vi "TOP-累积剂量数据管理.vi"(8 "错误输出":errorcluster, 11 "DB动作集":T1) -> (0 "error out":errorcluster, 3 "输出数据":variant)   [LabVIEW 2017]
uses:
  <vilib>/addons/database/Connection.llb/Conn ObjectReference.ctl
  <vilib>/addons/database/NI_Database_API.lvlib
panel:
  out "累积记录":T3
  out "探测器信息":T4
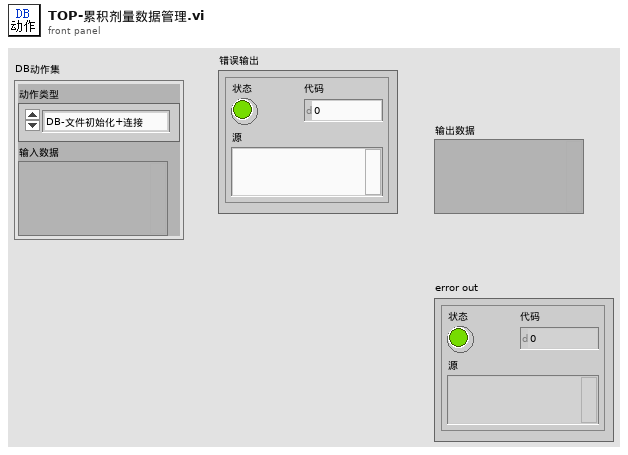
[diagram p1: front panel]
types:
  T1 = typedef "DB动作与数据.ctl" = cluster{"动作类型":T2, "输入数据":variant}
  T2 = typedef "DB动作类型.ctl" = enum16{"DB-文件初始化+连接", "DB-断开连接", "DB-结构初始化", "DB-加载设备", "DB-检查连接状态", "设备-登记新设备+数据表", "设备-删除设备", "设备-修改网址", "设备-修改名称+转移数据", "设备-修改备注", "设备-修改限值", "设备-累积校准", "设备-重排", "数据-获取全部", "数据-删除数据", "数据-写改累积记录+改累积剂量", "读变量-全部设备"}
  T3 = typedef "单条累积记录.ctl" = cluster{"起始时间":timestamp, "结束时间":timestamp, "累积剂量":dbl}
  T4 = typedef "探测器信息.ctl" = cluster{"网络地址":string, "名称":string, "备注":string, "累积剂量":dbl, "累积限值":dbl, "硬件剂量率限值":T5, "剂量率限值1":dbl, "剂量率限值2":dbl, "报警方式":T6}
  T5 = typedef "探头剂量率限值选择.ctl" = enum16{"一级限值", "二级限值"}
  T6 = typedef "报警方式选择.ctl" = enum16{"常报警", "自动静音", "手动静音"}
  T7 = typedef "修改网址.ctl" = cluster{"探头属性":T4, "新网址":string}
  T8 = typedef "设备改名卡.ctl" = cluster{"原名":string, "新名":string}
  T9 = typedef "删除记录输入.ctl" = cluster{"名称":string, "多条记录(空则全删)":T3[]}
  T10 = typedef "写改累积记录输入.ctl" = cluster{"探头地址与信息":T4, "测量值":T11, "累积记录":T3}
  T11 = typedef "测量值.ctl" = cluster{"时间":timestamp, "数值":dbl}
  T12 = typedef "NI_Database_API.lvlib/Conn ObjectReference.ctl" = refnum<k1>
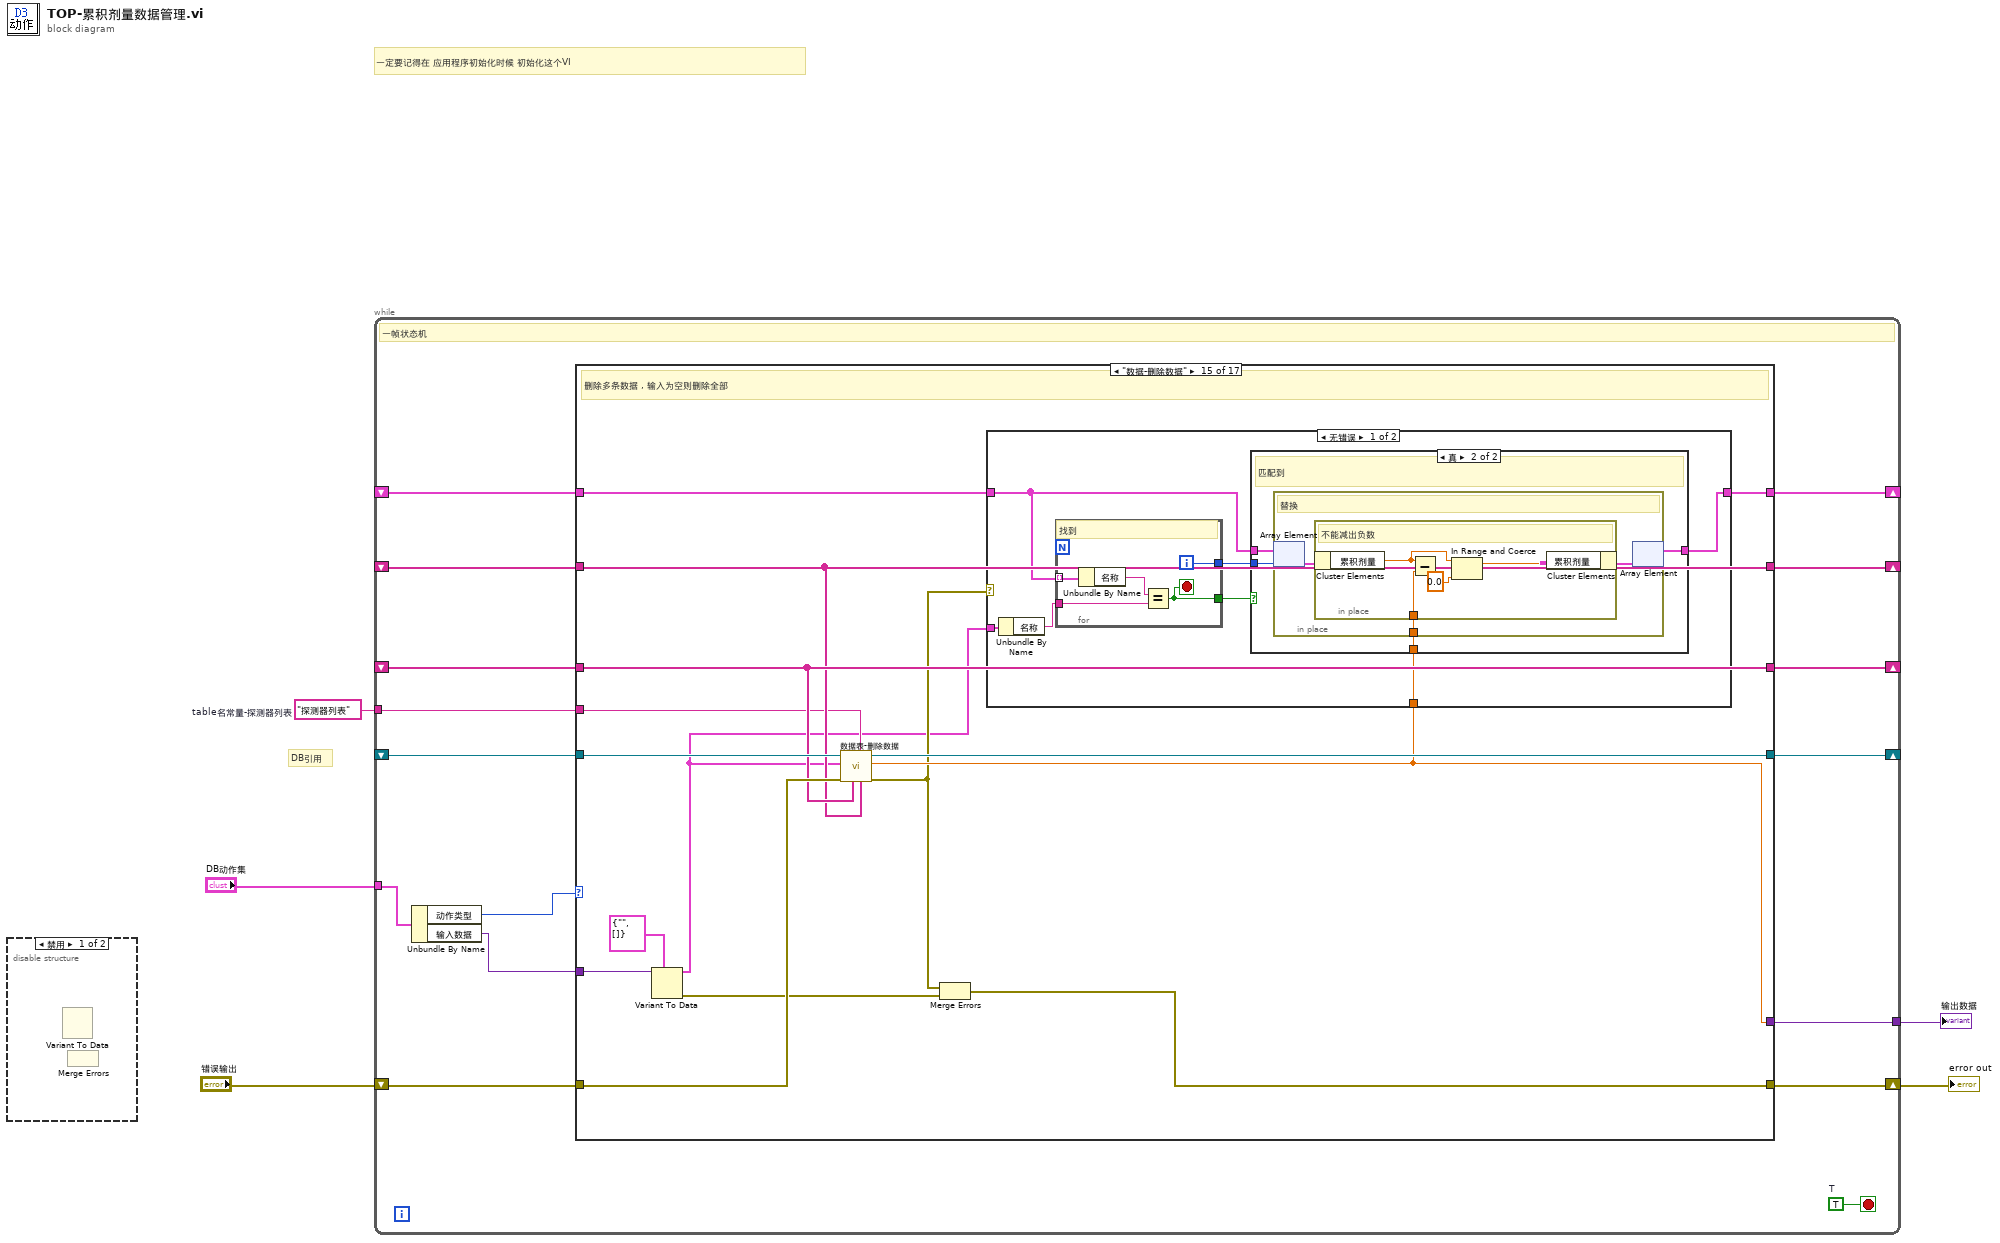
[diagram p0: block diagram]
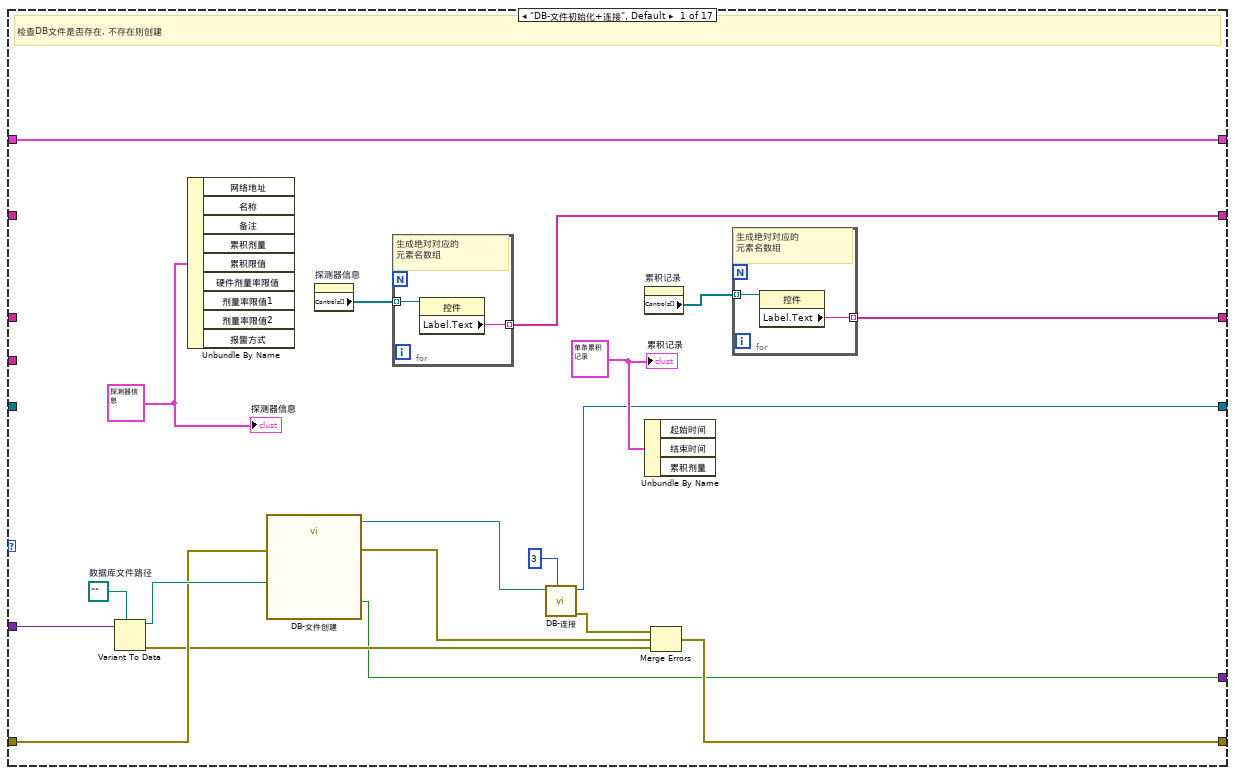
[diagram p3: hidden frame]
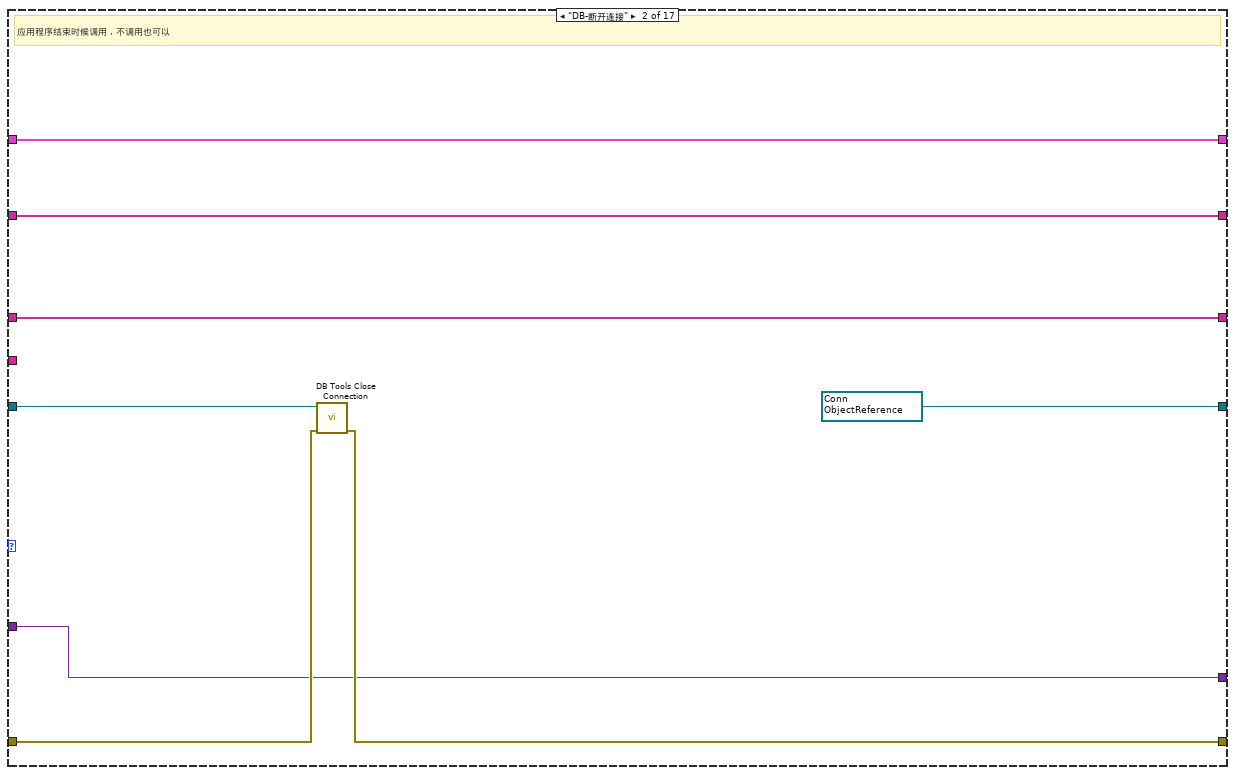
[diagram p4: hidden frame]
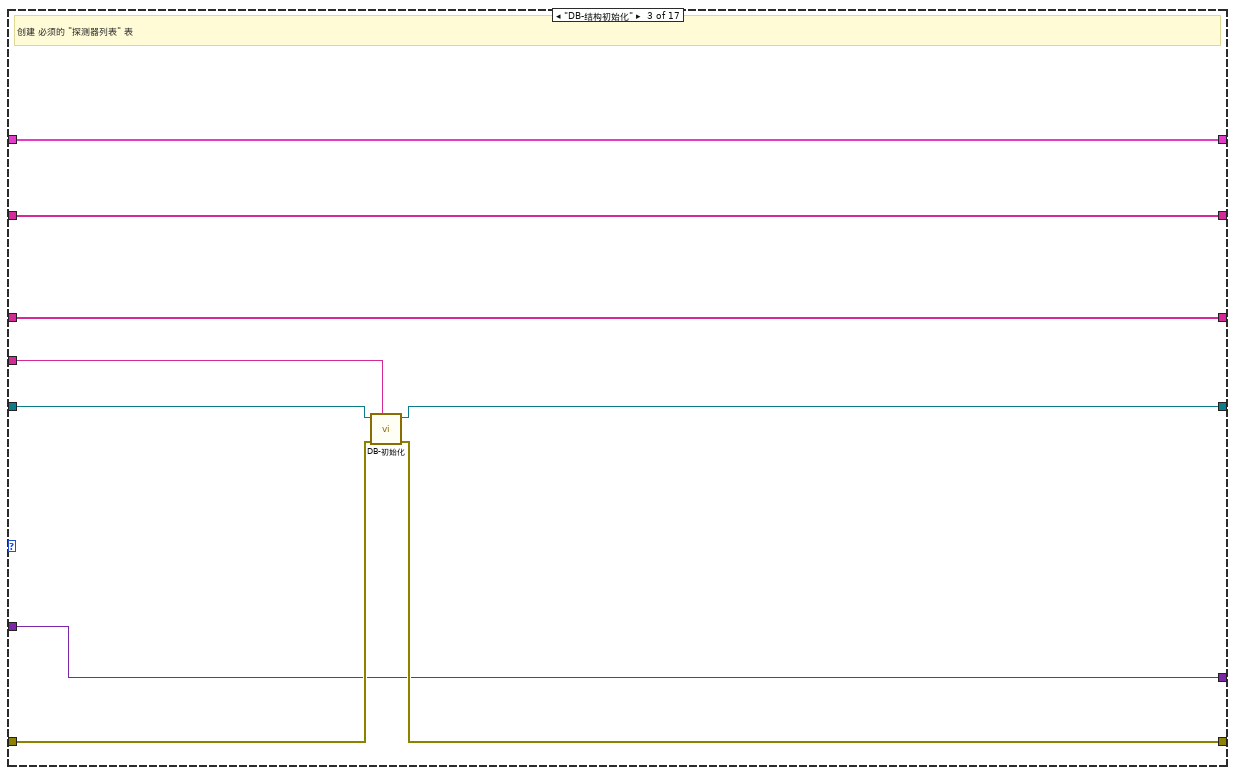
[diagram p5: hidden frame]
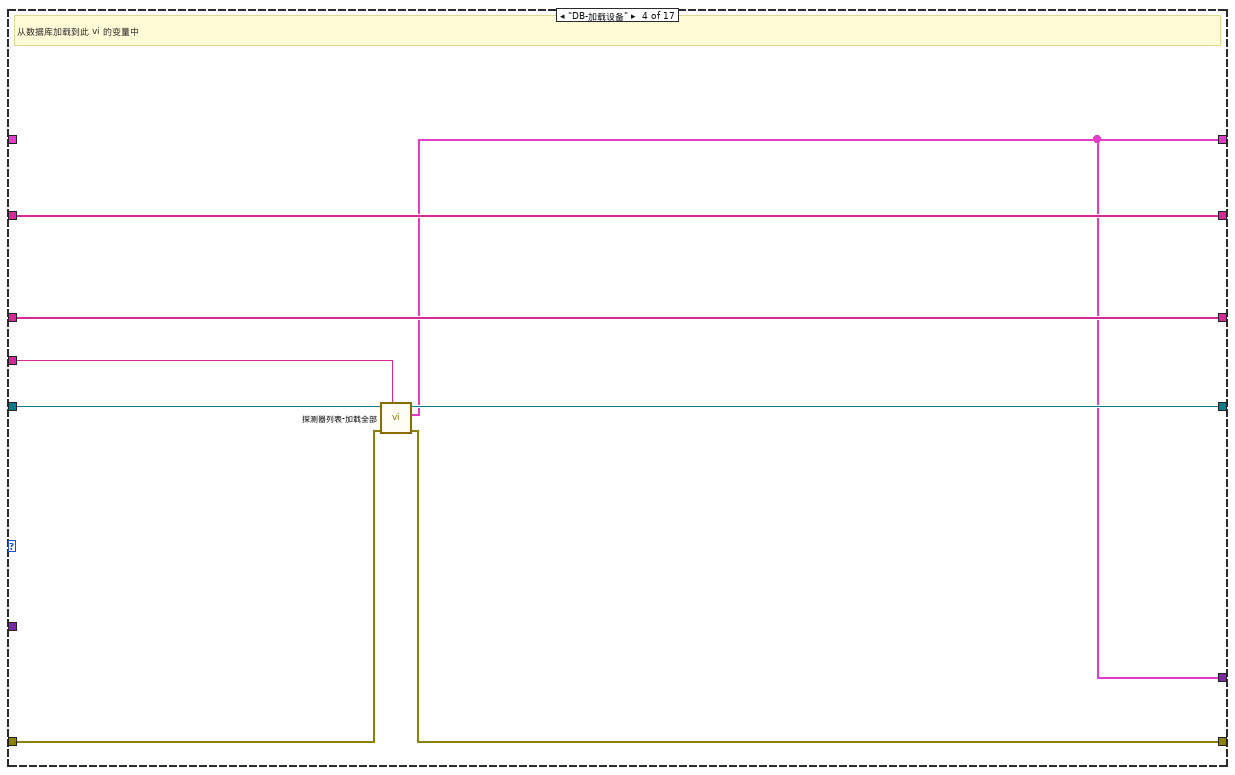
[diagram p6: hidden frame]
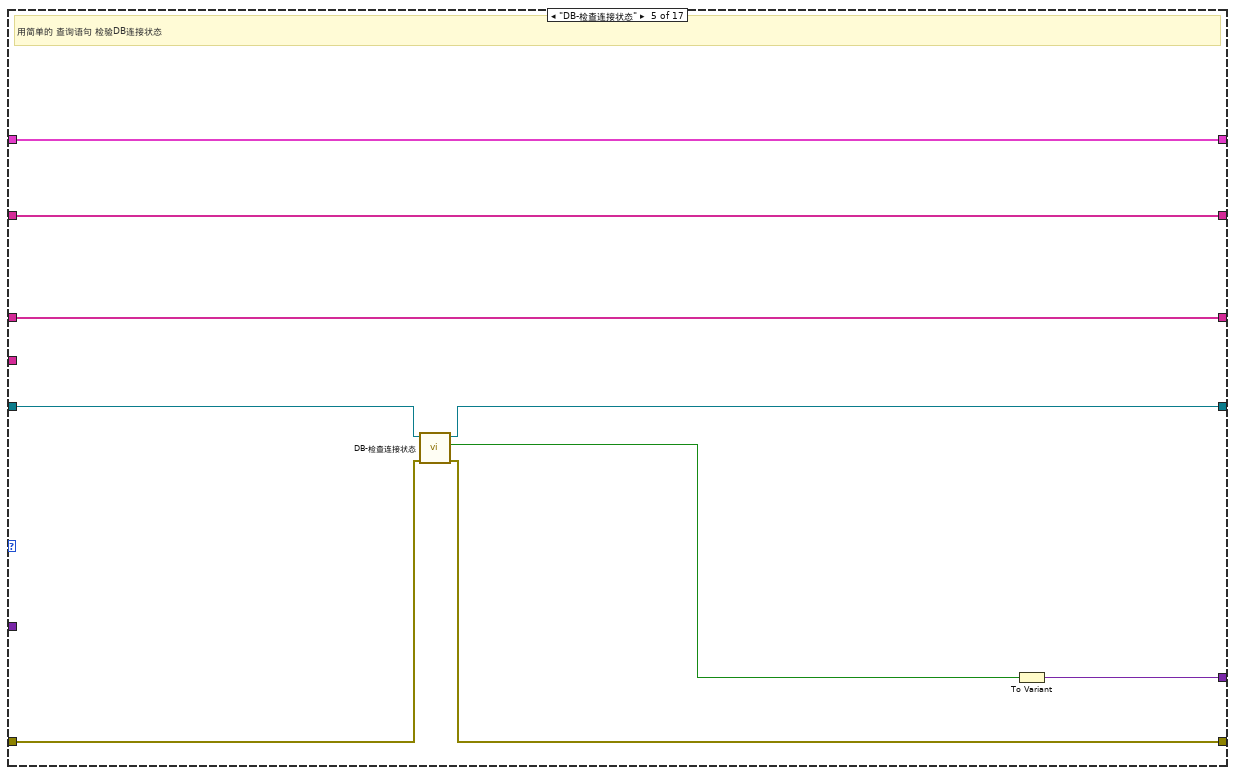
[diagram p7: hidden frame]
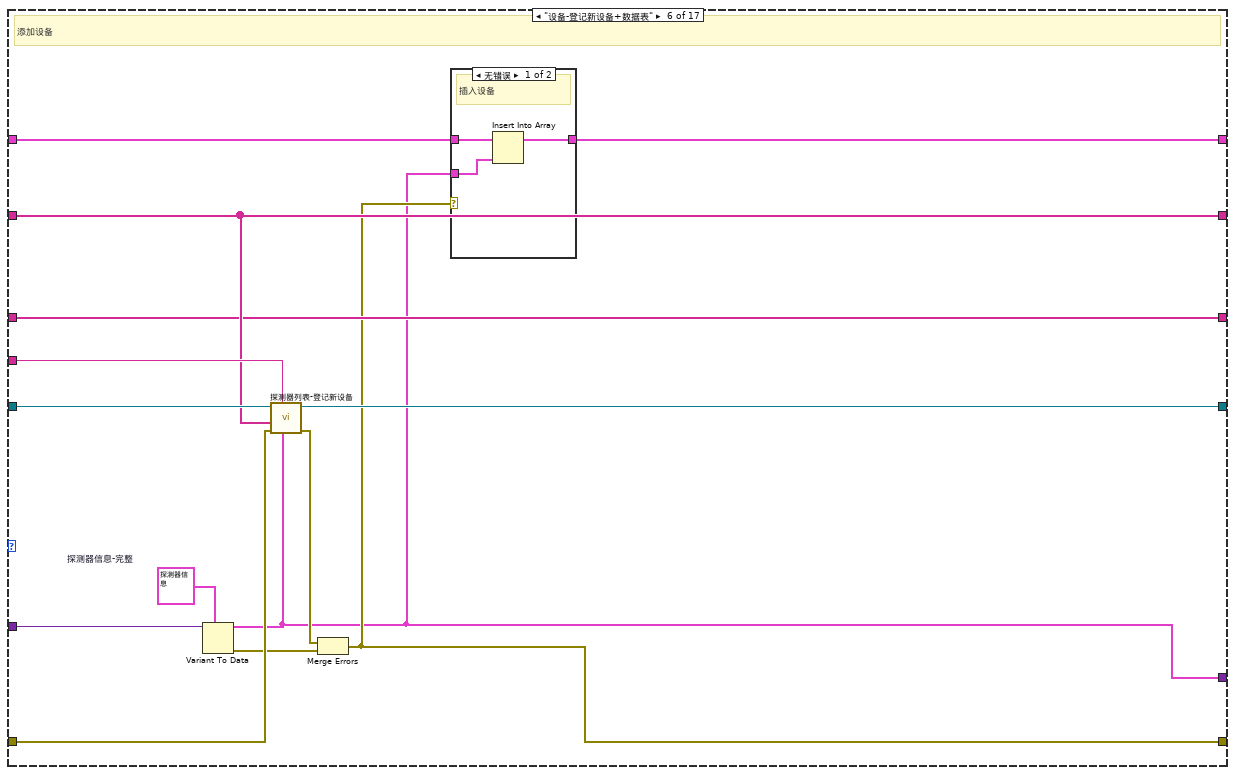
[diagram p8: hidden frame]
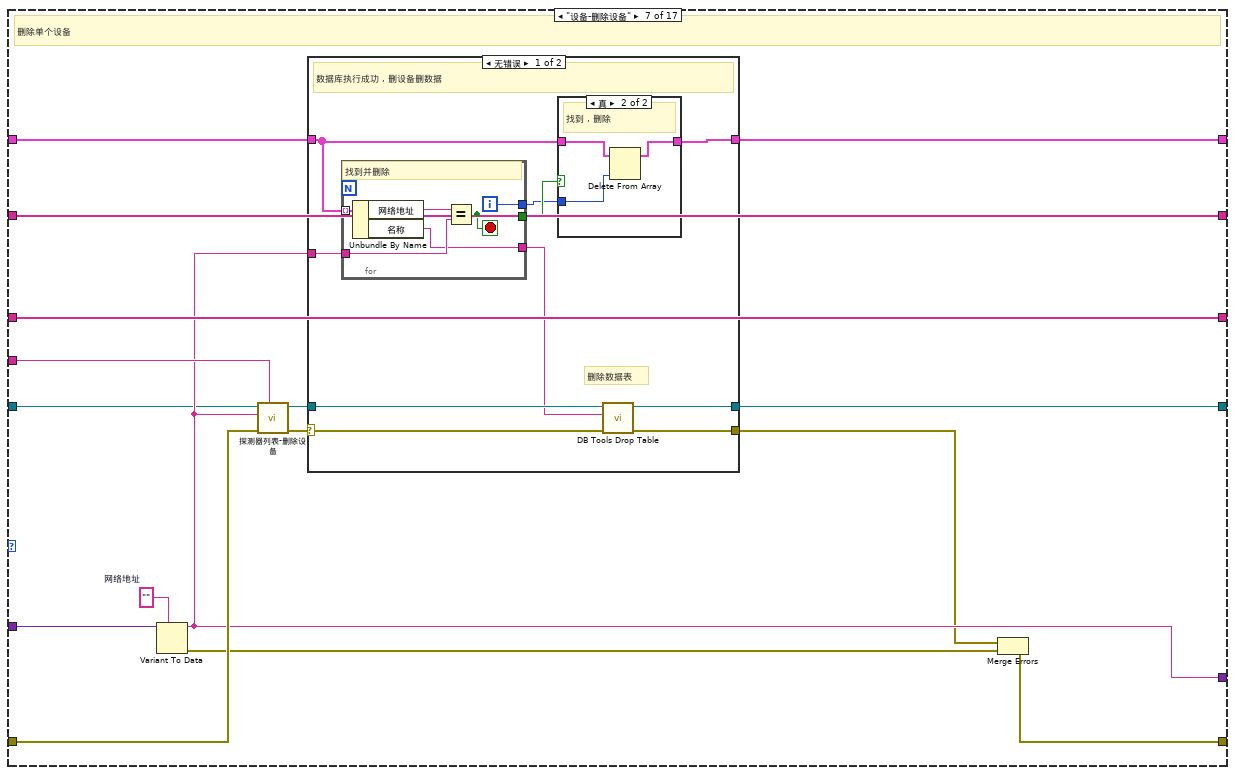
[diagram p10: hidden frame]
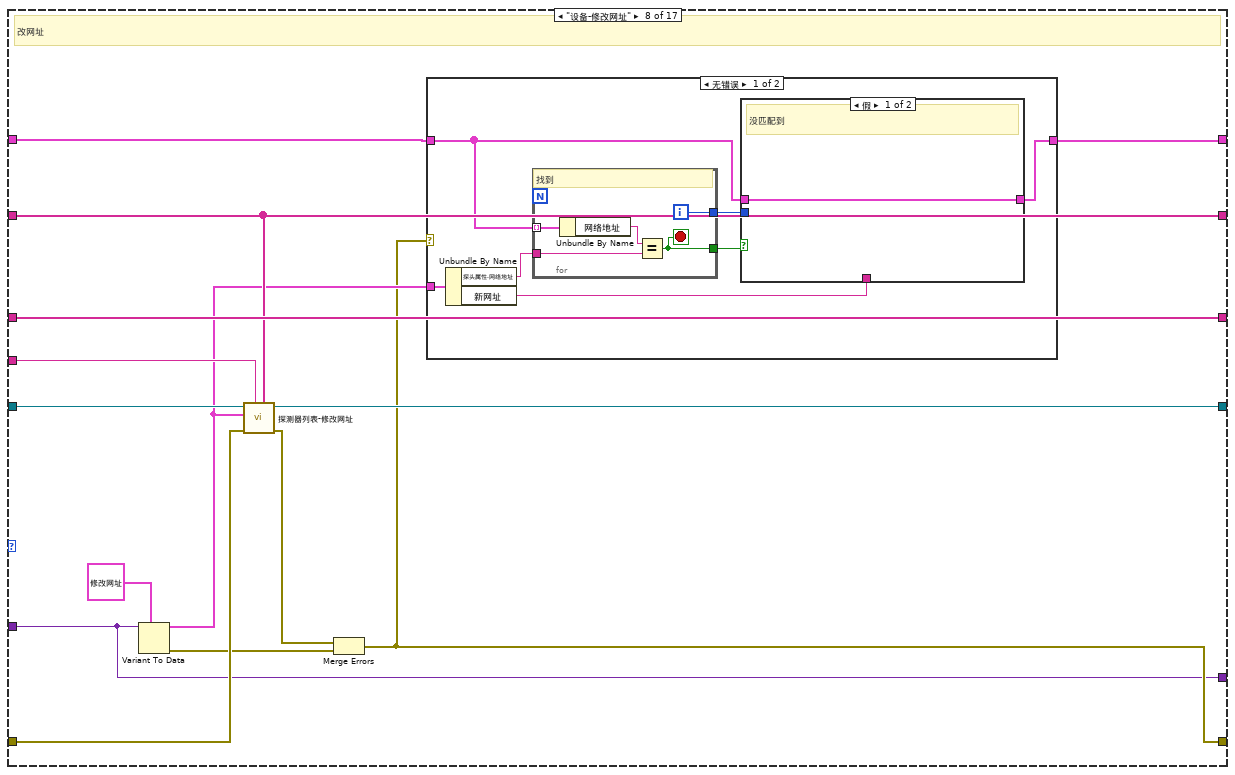
[diagram p13: hidden frame]
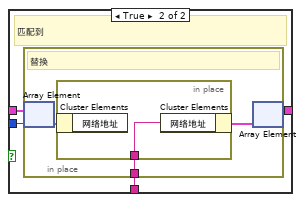
[diagram p14: hidden frame]
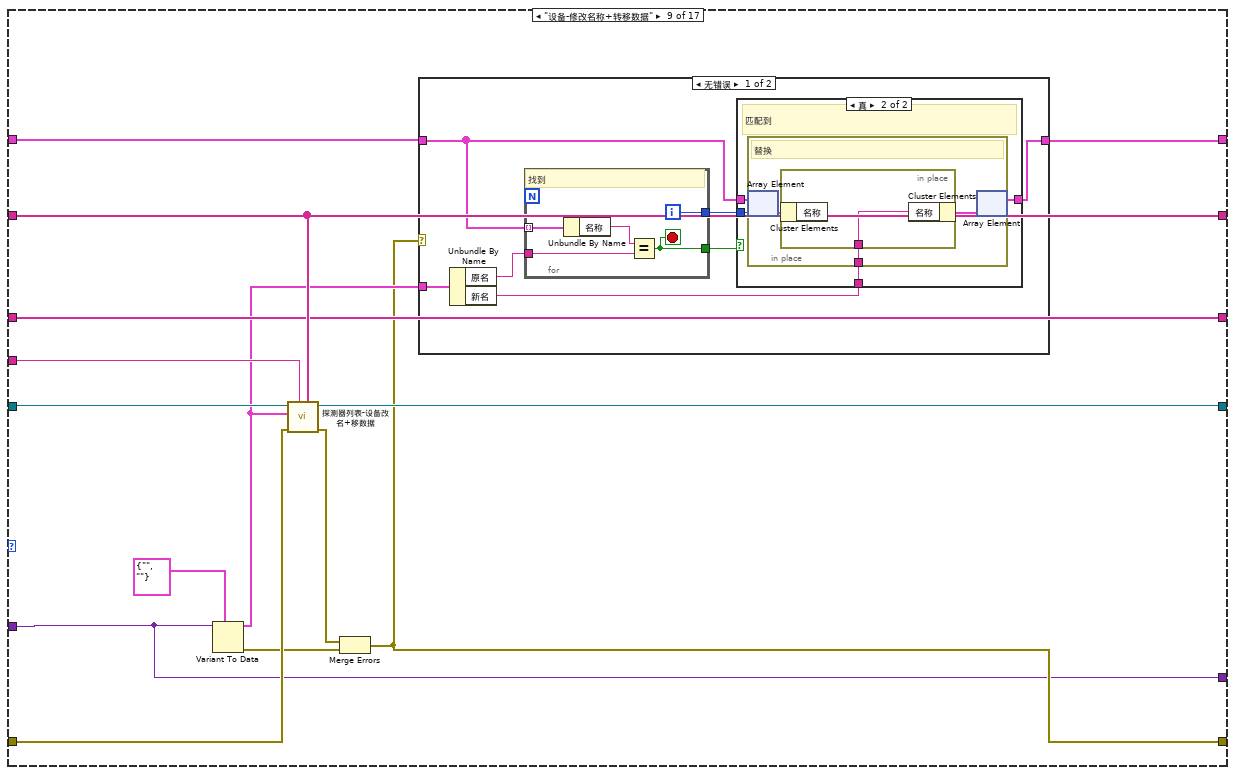
[diagram p16: hidden frame]
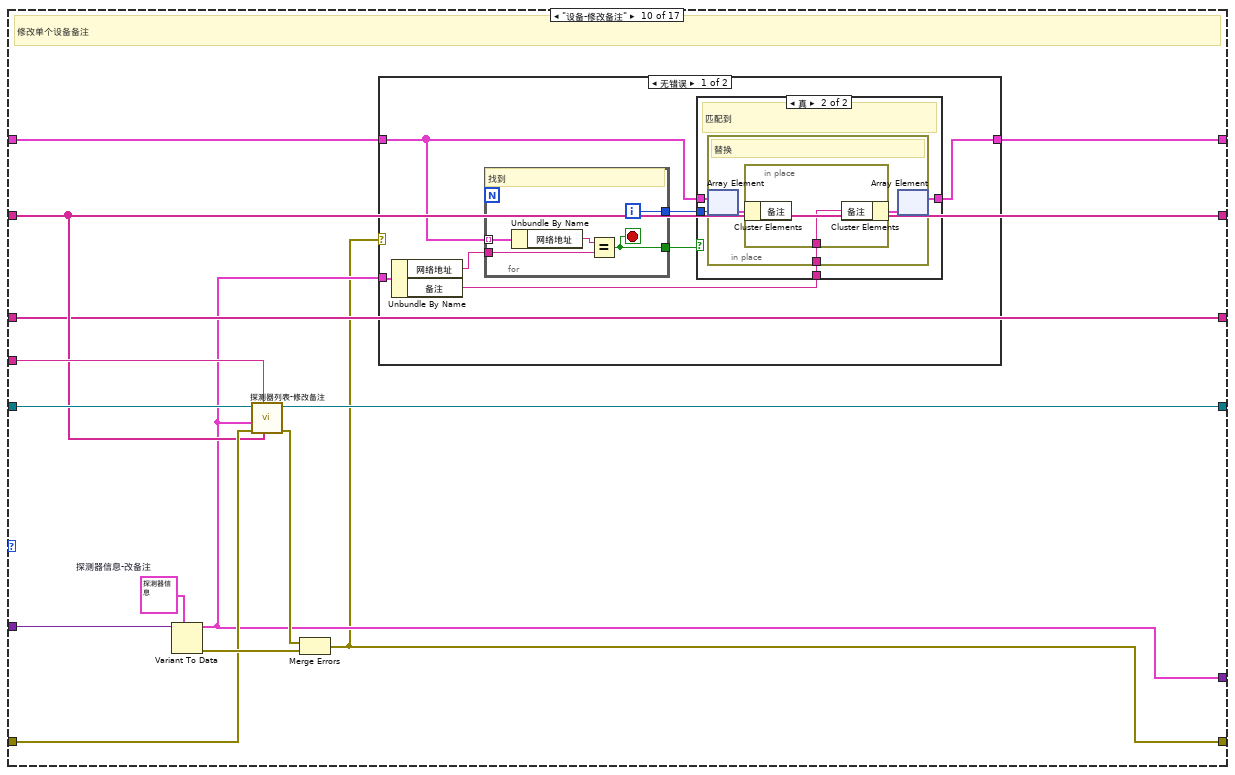
[diagram p19: hidden frame]
diagram:
  w4 = "探测器列表"  # table名常量-探测器列表
  # "DB引用"
  # "一定要记得在 应用程序初始化时候 初始化这个VI"
  n1 = disable-structure shown="禁用" {
    frame Disabled {
      n2 = Variant To Data() -> ()  [unwired: 3 in, 2 out]
      n3 = Merge Errors() -> ()  [unwired: 2 in, 1 out]
    }
    frame Enabled {
    }
  }
  n4 = while {
    shift-right: [w20] -> _
    shift-left: _ -> [w19]
    shift-right: [w7] -> w2
    shift-left: "错误输出" -> [w21]
    tunnel: w4 -> [w18]
    tunnel: [w17] -> w3
    shift-right: [w11] -> _
    shift-left: _ -> [w16]
    shift-right: [w12] -> _
    shift-left: _ -> [w15]
    shift-right: [w10] -> _
    shift-left: _ -> [w9]
    tunnel: "DB动作集" -> [w8]
    stop <- w6 stop-if-true
    w6 = TRUE  # T
    # "一帧状态机"
    n5 = Unbundle By Name(w8) -> ("动作类型"=w14:T2, "输入数据"=w13:variant)
    n6 = case shown="\"数据-删除数据\"" w14 {
      tunnel: w13 -> [w40 w48 w56 _ _ w88 w110 w136 w172 w218 w254 w295 w331 w343 w358 w398 _]
      tunnel: w21 -> [w37 w51 w59 w67 w76 w89 w111 w146 w183 w215 w251 w296 w323 w344 w359 w401 w432]
      tunnel: [w36 w50 w57 w66 w75 w80 w107 w137 w173 w209 w244 w289 w322 w338 w356 w388 w432] -> w7
      tunnel: [w25 w49 w58 w65 w77 w91 w98 w147 w180 w220 w256 w297 w324 w345 w360 w402 w431] -> w20
      tunnel: w19 -> [_ w52 w60 w69 w78 w92 w100 w149 w185 w221 w257 w298 w332 w346 w361 w403 w431]
      tunnel: w18 -> [_ _ w61 w68 _ w90 w112 w142 w181 w219 w255 w293 w333 _ w353 w394 _]
      tunnel: [w22 w48 w56 w62 w73 w79 w102 w136 w172 w210 w245 w284 w320 w337 w350 w389 w428] -> w17
      tunnel: w16 -> [_ w47 w55 w64 w72 w84 w106 w141 w178 w214 w249 w286 w326 w336 w354 w395 w430]
      tunnel: w15 -> [_ w46 w54 w63 w71 w83 w105 w143 w177 w213 w248 w285 w325 w335 w355 w397 w429]
      tunnel: [w33 w46 w54 w63 w71 w83 w105 w143 w177 w213 w248 w285 w325 w335 w355 w397 w429] -> w12
      tunnel: [w31 w47 w55 w64 w72 w84 w106 w141 w178 w214 w249 w286 w326 w336 w354 w395 w430] -> w11
      tunnel: [w30 w45 w53 w62 w70 w81 w101 w139 w175 w208 w246 w287 w327 w334 w347 w392 w428] -> w10
      tunnel: w9 -> [w30 w45 w53 _ w70 w82 w103 w140 w176 w211 w247 w290 w328 w334 w351 w393 w428]
      frame "DB-文件初始化+连接", Default {
        w28 = T3 {"起始时间"=timestamp(0 s since 1904-01-01), "结束时间"=timestamp(0 s since 1904-01-01), "累积剂量"=0.0} ("累积记录")
        w29 = T4 {"网络地址"="", "名称"="", "备注"="", "累积剂量"=0.0, "累积限值"=0.0, "硬件剂量率限值"=enum."一级限值", "剂量率限值1"=0.0, "剂量率限值2"=0.0, "报警方式"=enum."常报警"} ("探测器信息")
        w39 = path ""  # 数据库文件路径
        # "检查DB文件是否存在, 不存在则创建"
        n7 = Variant To Data(type=w39, Variant=w40) -> (data=w38:path, error out=w35:errorcluster)  [unwired: 1 in]
        n8 = Unbundle By Name(w29) -> ()  [unwired: 9 out]
        n9 = call "DB-文件创建.vi"("错误常量"=w37, "文件路径输入控件"=w38) -> ("错误输出"=w23:errorcluster, "已存在？"=w22:bool, "DB路径 o"=w26:path)  [unwired: 7 in]
        n10 = property on="探测器信息" class="簇 (严格)"() -> ("Controls[]"=w32:refnum<vi>[])  [unwired: 2 in, 2 out]
        n11 = for {
          tunnel: w32 -> [w42] mode=indexing
          tunnel: [w41] -> w31 mode=indexing
          # "生成绝对对应的\n元素名数组"
          n12 = property class="控件"(reference=w42) -> ("Label.Text"=w41:string)  [unwired: 1 in, 2 out]
        }
        n13 = call "DB-连接.vi"("超时(5)"=3, "DB路径"=w26) -> ("error out"=w24:errorcluster, "connection reference"=w25:T12)  [unwired: 8 in]
        n14 = property on="累积记录" class="簇 (严格)"() -> ("Controls[]"=w34:refnum<vi>[])  [unwired: 2 in, 2 out]
        n15 = Unbundle By Name(w28) -> ()  [unwired: 3 out]
        n16 = Merge Errors(w24, w23, w35) -> (w36:errorcluster)
        n17 = for {
          tunnel: w34 -> [w44] mode=indexing
          tunnel: [w43] -> w33 mode=indexing
          # "生成绝对对应的\n元素名数组"
          n18 = property class="控件"(reference=w44) -> ("Label.Text"=w43:string)  [unwired: 1 in, 2 out]
        }
        "累积记录" <- w28
        "探测器信息" <- w29
      }
      frame "DB-断开连接" {
        w49 = T12 refnum items=["Connection"] ("connection reference out")
        # "应用程序结束时候调用 , 不调用也可以"
        n19 = call <vilib>:"DB Tools Close Connection.vi"("error in (no error)"=w51, "connection reference"=w52) -> ("error out"=w50:errorcluster)  [unwired: 5 in]
      }
      frame "DB-结构初始化" {
        # "创建 必须的 \"探测器列表\" 表"
        n20 = call "DB-初始化.vi"("table-探测器列表名"=w61, "error in (no error)"=w59, "数据库引用"=w60) -> ("error out"=w57:errorcluster, "connection reference out"=w58:T12)  [unwired: 7 in]
      }
      frame "DB-加载设备" {
        # "从数据库加载到此 vi 的变量中"
        n21 = call "探测器列表-加载全部.vi"("table-探测器列表名"=w68, "error in (no error)"=w67, "数据库引用"=w69) -> ("error out"=w66:errorcluster, "探测器清单"=w62:T4[], "connection reference out"=w65:T12)  [unwired: 6 in]
      }
      frame "DB-检查连接状态" {
        # "用简单的 查询语句 检验DB连接状态"
        n22 = call "DB-检查连接状态.vi"("error in (no error)"=w76, "数据库引用"=w78) -> ("error out"=w75:errorcluster, "连接正常?"=w74:bool, "数据库连接引用out"=w77:T12)  [unwired: 7 in]
        n23 = To Variant(anything=w74) -> (Variant=w73:variant)
      }
      frame "设备-登记新设备+数据表" {
        w87 = T4 {"网络地址"="", "名称"="", "备注"="", "累积剂量"=0.0, "累积限值"=0.0, "硬件剂量率限值"=enum."一级限值", "剂量率限值1"=0.0, "剂量率限值2"=0.0, "报警方式"=enum."常报警"}  # 探测器信息-完整
        # "添加设备"
        n24 = Variant To Data(type=w87, Variant=w88) -> (data=w79:T4, error out=w86:errorcluster)  [unwired: 1 in]
        n25 = call "探测器列表-登记新设备.vi"("探测器信息"=w79, "table-探测器列表名"=w90, "error in (no error)"=w89, "元素名[]-探测器信息"=w84, "数据库引用"=w92) -> ("error out"=w85:errorcluster, "connection reference out"=w91:T12)  [unwired: 5 in]
        n26 = Merge Errors(w85, w86) -> (w80:errorcluster)
        n27 = case shown="无错误" w80 {
          tunnel: w82 -> [w95 w96]
          tunnel: w79 -> [w94 _]
          tunnel: [w93 w96] -> w81
          frame No Error {
            # "插入设备"
            n28 = Insert Into Array(array=w95, new element=w94) -> (w93:T4[])  [unwired: 1 in]
          }
          frame Error {
          }
        }
      }
      frame "设备-删除设备" {
        w109 = ""  # 网络地址
        # "删除单个设备"
        n29 = Variant To Data(type=w109, Variant=w110) -> (data=w102:string, error out=w108:errorcluster)  [unwired: 1 in]
        n30 = call "探测器列表-删除设备.vi"("table名-探测器列表"=w112, "error in (no error)"=w111, "网络地址"=w102, "数据库引用"=w100) -> ("error out"=w104:errorcluster, "connection reference out"=w99:T12)  [unwired: 6 in]
        n31 = case shown="无错误" w104 {
          selector: w104 -> [w115 w133]
          tunnel: w103 -> [w119 w135]
          tunnel: w102 -> [w122 _]
          tunnel: [w118 w135] -> w101
          tunnel: w99 -> [w117 w134]
          tunnel: [w114 w134] -> w98
          tunnel: [w113 w133] -> w97
          frame No Error {
            # "删除数据表"
            # "数据库执行成功 , 删设备删数据"
            n32 = for {
              tunnel: w119 -> [w128] mode=indexing
              tunnel: w122 -> [w131]
              tunnel: [w130] -> w120
              tunnel: [w129] -> w121
              tunnel: [w127] -> w116
              i -> [w130]
              stop <- w129 stop-if-true
              # "找到并删除"
              n33 = Unbundle By Name(w128) -> ("网络地址"=w132:string, "名称"=w127:string)
              n34 = Equal?(x=w132, y=w131) -> (x = y?=w129:bool)
            }
            n35 = case shown="真" w121 {
              tunnel: w120 -> [_ w125]
              tunnel: w119 -> [w123 w126]
              tunnel: [w123 w124] -> w118
              frame False {
              }
              frame True {
                # "找到 , 删除"
                n36 = Delete From Array(array=w126, index=w125) -> (array with subset deleted=w124:T4[])  [unwired: 1 in, 1 out]
              }
            }
            n37 = call <vilib>:"DB Tools Drop Table.vi"("error in (no error)"=w115, "table"=w116, "connection reference"=w117) -> ("error out"=w113:errorcluster, "connection reference out"=w114:T12)  [unwired: 5 in]
          }
          frame Error {
            # "数据库执行失败"
          }
        }
        n38 = Merge Errors(w97, w108) -> (w107:errorcluster)
      }
      frame "设备-修改网址" {
        # "改网址"
        n39 = Variant To Data(type=T7 {"探头属性"={"网络地址"="", "名称"="", "备注"="", "累积剂量"=0.0, "累积限值"=0.0, "硬件剂量率限值"=enum."一级限值", "剂量率限值1"=0.0, "剂量率限值2"=0.0, "报警方式"=enum."常报警"}, "新网址"=""} ("类型"), Variant=w136) -> (data=w138:T7, error out=w145:errorcluster)  [unwired: 1 in]
        n40 = call "探测器列表-修改网址.vi"("元素名[]-探测器信息"=w141, "table名-探测器列表"=w142, "error in (no error)"=w146, "修改网址"=w138, "数据库引用"=w149) -> ("error out"=w144:errorcluster, "数据库连接引用out"=w147:T12)  [unwired: 5 in]
        n41 = Merge Errors(w144, w145) -> (w137:errorcluster)
        n42 = case shown="无错误" w137 {
          tunnel: w140 -> [w154 w171]
          tunnel: w138 -> [w156 _]
          tunnel: [w152 w171] -> w139
          frame No Error {
            n43 = Unbundle By Name(w156) -> ("探头属性.网络地址"=w155:string, "新网址"=w151:string)
            n44 = for {
              tunnel: w154 -> [w166] mode=indexing
              tunnel: w155 -> [w169]
              tunnel: [w168] -> w153
              tunnel: [w167] -> w150
              i -> [w168]
              stop <- w167 stop-if-true
              # "找到"
              n45 = Unbundle By Name(w166) -> ("网络地址"=w170:string)
              n46 = Equal?(x=w170, y=w169) -> (x = y?=w167:bool)
            }
            n47 = case shown="假" w150 {
              tunnel: w154 -> [w157 w161]
              tunnel: w153 -> [_ w160]
              tunnel: [w157 w159] -> w152
              tunnel: w151 -> [_ w158]
              frame False {
                # "没匹配到"
              }
              frame True {
                # "匹配到"
                n48 = in-place {
                  in-place-border: w158 -> [w163]
                  # "替换"
                  n49 = in-place-array #1(w161, w160) -> (w164:T4)
                  n50 = in-place {
                    in-place-border: w163 -> [w165]
                    n51 = in-place-cluster #2(w164) -> ()  [unwired: 1 out]
                    n52 = in-place-cluster #2("网络地址"=w165) -> (w162:T4)
                  }
                  n53 = in-place-array #1(w162) -> (w159:T4[])  [unwired: 1 out]
                }
              }
            }
          }
          frame Error {
          }
        }
      }
      frame "设备-修改名称+转移数据" {
        n54 = Variant To Data(type=T8 {"原名"="", "新名"=""} ("改名"), Variant=w172) -> (data=w174:T8, error out=w182:errorcluster)  [unwired: 1 in]
        n55 = call "探测器列表-设备改名+移数据.vi"("元素名[]-探测器信息"=w178, "table名-探测器列表"=w181, "error in (no error)"=w183, "改名"=w174, "数据库引用"=w185) -> ("error out"=w179:errorcluster, "数据库连接引用out"=w180:T12)  [unwired: 5 in]
        n56 = Merge Errors(w179, w182) -> (w173:errorcluster)
        n57 = case shown="无错误" w173 {
          tunnel: w176 -> [w190 w207]
          tunnel: w174 -> [w192 _]
          tunnel: [w188 w207] -> w175
          frame No Error {
            n58 = Unbundle By Name(w192) -> ("原名"=w191:string, "新名"=w187:string)
            n59 = for {
              tunnel: w190 -> [w202] mode=indexing
              tunnel: w191 -> [w205]
              tunnel: [w204] -> w189
              tunnel: [w203] -> w186
              i -> [w204]
              stop <- w203 stop-if-true
              # "找到"
              n60 = Unbundle By Name(w202) -> ("名称"=w206:string)
              n61 = Equal?(x=w206, y=w205) -> (x = y?=w203:bool)
            }
            n62 = case shown="真" w186 {
              tunnel: w190 -> [w193 w197]
              tunnel: w189 -> [_ w196]
              tunnel: [w193 w195] -> w188
              tunnel: w187 -> [_ w194]
              frame False {
                # "没匹配到"
              }
              frame True {
                # "匹配到"
                n63 = in-place {
                  in-place-border: w194 -> [w199]
                  # "替换"
                  n64 = in-place-array #3(w197, w196) -> (w200:T4)
                  n65 = in-place {
                    in-place-border: w199 -> [w201]
                    n66 = in-place-cluster #4(w200) -> ()  [unwired: 1 out]
                    n67 = in-place-cluster #4("名称"=w201) -> (w198:T4)
                  }
                  n68 = in-place-array #3(w198) -> (w195:T4[])  [unwired: 1 out]
                }
              }
            }
          }
          frame Error {
          }
        }
      }
      frame "设备-修改备注" {
        w217 = T4 {"网络地址"="", "名称"="", "备注"="", "累积剂量"=0.0, "累积限值"=0.0, "硬件剂量率限值"=enum."一级限值", "剂量率限值1"=0.0, "剂量率限值2"=0.0, "报警方式"=enum."常报警"}  # 探测器信息-改备注
        # "修改单个设备备注"
        n69 = Variant To Data(type=w217, Variant=w218) -> (data=w210:T4, error out=w216:errorcluster)  [unwired: 1 in]
        n70 = call "探测器列表-修改备注.vi"("元素名[]-探测器信息"=w214, "table名-探测器列表"=w219, "error in (no error)"=w215, "探测器信息"=w210, "数据库引用"=w221) -> ("error out"=w212:errorcluster, "connection reference out"=w220:T12)  [unwired: 5 in]
        n71 = Merge Errors(w212, w216) -> (w209:errorcluster)
        n72 = case shown="无错误" w209 {
          tunnel: w211 -> [w226 w243]
          tunnel: w210 -> [w228 _]
          tunnel: [w223 w243] -> w208
          frame No Error {
            n73 = Unbundle By Name(w228) -> ("网络地址"=w227:string, "备注"=w224:string)
            n74 = for {
              tunnel: w226 -> [w238] mode=indexing
              tunnel: w227 -> [w241]
              tunnel: [w240] -> w225
              tunnel: [w239] -> w222
              i -> [w240]
              stop <- w239 stop-if-true
              # "找到"
              n75 = Unbundle By Name(w238) -> ("网络地址"=w242:string)
              n76 = Equal?(x=w242, y=w241) -> (x = y?=w239:bool)
            }
            n77 = case shown="真" w222 {
              tunnel: w226 -> [w229 w233]
              tunnel: w225 -> [_ w232]
              tunnel: w224 -> [_ w231]
              tunnel: [w229 w230] -> w223
              frame False {
                # "没匹配到"
              }
              frame True {
                # "匹配到"
                n78 = in-place {
                  in-place-border: w231 -> [w235]
                  # "替换"
                  n79 = in-place-array #5(w233, w232) -> (w236:T4)
                  n80 = in-place {
                    in-place-border: w235 -> [w237]
                    n81 = in-place-cluster #6(w236) -> ()  [unwired: 1 out]
                    n82 = in-place-cluster #6("备注"=w237) -> (w234:T4)
                  }
                  n83 = in-place-array #5(w234) -> (w230:T4[])  [unwired: 1 out]
                }
              }
            }
          }
          frame Error {
          }
        }
      }
      frame "设备-修改限值" {
        w253 = T4 {"网络地址"="", "名称"="", "备注"="", "累积剂量"=0.0, "累积限值"=0.0, "硬件剂量率限值"=enum."一级限值", "剂量率限值1"=0.0, "剂量率限值2"=0.0, "报警方式"=enum."常报警"}  # 探测器信息-改限值
        # "修改单个设备的限值"
        n84 = Variant To Data(type=w253, Variant=w254) -> (data=w245:T4, error out=w252:errorcluster)  [unwired: 1 in]
        n85 = call "探测器列表-修改限值.vi"("元素名[]-探测器信息"=w249, "table名-探测器列表"=w255, "error in (no error)"=w251, "探测器信息"=w245, "数据库引用"=w257) -> ("error out"=w250:errorcluster, "connection reference out"=w256:T12)  [unwired: 5 in]
        n86 = Merge Errors(w250, w252) -> (w244:errorcluster)
        n87 = case shown="无错误" w244 {
          tunnel: w247 -> [w262 w283]
          tunnel: w245 -> [w259 _]
          tunnel: [w260 w283] -> w246
          frame No Error {
            n88 = Unbundle By Name(w259) -> ("网络地址"=w263:string)
            n89 = for {
              tunnel: w262 -> [w278] mode=indexing
              tunnel: w263 -> [w281]
              tunnel: [w280] -> w261
              tunnel: [w279] -> w258
              i -> [w280]
              stop <- w279 stop-if-true
              # "找到"
              n90 = Unbundle By Name(w278) -> ("网络地址"=w282:string)
              n91 = Equal?(x=w282, y=w281) -> (x = y?=w279:bool)
            }
            n92 = case shown="真" w258 {
              tunnel: w262 -> [w264 w268]
              tunnel: w261 -> [_ w267]
              tunnel: [w264 w266] -> w260
              tunnel: w259 -> [_ w265]
              frame False {
                # "没匹配到"
              }
              frame True {
                # "匹配到"
                n93 = in-place {
                  in-place-border: w265 -> [w269]
                  # "替换"
                  n94 = in-place-array #7(w268, w267) -> (w271:T4)
                  n95 = in-place {
                    in-place-border: w269 -> [w277]
                    n96 = in-place-cluster #8(w271) -> ()  [unwired: 5 out]
                    n97 = Unbundle By Name(w277) -> ("累积限值"=w276:dbl, "硬件剂量率限值"=w275:T5, "剂量率限值1"=w274:dbl, "剂量率限值2"=w273:dbl, "报警方式"=w272:T6)
                    n98 = in-place-cluster #8("累积限值"=w276, "硬件剂量率限值"=w275, "剂量率限值1"=w274, "剂量率限值2"=w273, "报警方式"=w272) -> (w270:T4)
                  }
                  n99 = in-place-array #7(w270) -> (w266:T4[])  [unwired: 1 out]
                }
              }
            }
          }
          frame Error {
          }
        }
      }
      frame "设备-累积校准" {
        w294 = ""  # 名称
        # "实时累积 或 删除部分累积记录 时\n会出现 \n总累积剂量 与 数据表的累计之和 不相同的情况\n可在 上线 或 掉线 或 删除数据 之后执行同步操作。"
        # "将总累积剂量 与 数据表的所有记录之和 同步，防止差异扩大"
        n100 = Variant To Data(type=w294, Variant=w295) -> (data=w288:string, error out=w291:errorcluster)  [unwired: 1 in]
        n101 = call "探测器列表-累积校准.vi"("元素名[]-探测器信息"=w286, "元素名[]-累积记录"=w285, "error in (no error)"=w296, "表名-设备表"=w293, "名称"=w288, "数据库引用"=w298) -> ("error out"=w292:errorcluster, "校准值"=w284:dbl, "connection reference out"=w297:T12)  [unwired: 3 in]
        n102 = Merge Errors(w292, w291) -> (w289:errorcluster)
        n103 = case shown="无错误" w289 {
          tunnel: w290 -> [w304 w319]
          tunnel: w288 -> [w299 _]
          tunnel: [w302 w319] -> w287
          tunnel: w284 -> [w301 _]
          frame No Error {
            n104 = for {
              tunnel: w304 -> [w314] mode=indexing
              tunnel: w299 -> [w317]
              tunnel: [w316] -> w303
              tunnel: [w315] -> w300
              i -> [w316]
              stop <- w315 stop-if-true
              # "找到"
              n105 = Unbundle By Name(w314) -> ("名称"=w318:string)
              n106 = Equal?(x=w318, y=w317) -> (x = y?=w315:bool)
            }
            n107 = case shown="真" w300 {
              tunnel: w304 -> [w305 w309]
              tunnel: w303 -> [_ w308]
              tunnel: [w305 w307] -> w302
              tunnel: w301 -> [_ w306]
              frame False {
                # "没匹配到"
              }
              frame True {
                # "匹配到"
                n108 = in-place {
                  in-place-border: w306 -> [w311]
                  # "替换"
                  n109 = in-place-array #9(w309, w308) -> (w312:T4)
                  n110 = in-place {
                    in-place-border: w311 -> [w313]
                    n111 = in-place-cluster #10(w312) -> ()  [unwired: 1 out]
                    n112 = in-place-cluster #10("累积剂量"=w313) -> (w310:T4)
                  }
                  n113 = in-place-array #9(w310) -> (w307:T4[])  [unwired: 1 out]
                }
              }
            }
          }
          frame Error {
          }
        }
      }
      frame "设备-重排" {
        w330 = i32[] []  # 新顺序
        # "清空设备列表, 按新顺序写入设备列表"
        n114 = Variant To Data(type=w330, Variant=w331) -> (data=w329:i32[], error out=w321:errorcluster)  [unwired: 1 in]
        n115 = call "探测器列表-重排设备.vi"("元素名[]-探测器信息"=w326, "table名-探测器列表"=w333, "error in (no error)"=w323, "新顺序"=w329, "探测器清单"=w328, "数据库引用"=w332) -> ("error out"=w320:errorcluster, "探测器清单 new"=w327:T4[], "connection reference out"=w324:T12)  [unwired: 3 in]
        n116 = Merge Errors(w320, w321) -> (w322:errorcluster)
      }
      frame "数据-获取全部" {
        w341 = ""  # 表名-设备名
        # "数据量应该不会太大"
        # "单个设备的全部记录 , 数据量应该不会太大 , 所依每次从数据库读取"
        n117 = Variant To Data(type=w341, Variant=w343) -> (data=w342:string, error out=w340:errorcluster)  [unwired: 1 in]
        n118 = call "数据表-获取全部.vi"("元素名[]-累积记录"=w335, "error in (no error)"=w344, "table"=w342, "数据库引用"=w346) -> ("error out"=w339:errorcluster, "累积记录数据"=w337:T3[], "connection reference out"=w345:T12)  [unwired: 5 in]
        n119 = Merge Errors(w339, w340) -> (w338:errorcluster)
      }
      frame "数据-删除数据" {
        # "删除多条数据 , 输入为空则删除全部"
        n120 = Variant To Data(type=T9 {"名称"="", "多条记录(空则全删)"=[]}, Variant=w358) -> (data=w348:T9, error out=w357:errorcluster)  [unwired: 1 in]
        n121 = call "数据表-删除数据.vi"("元素名[]-探测器列表"=w354, "表名-设备表"=w353, "元素名[]-累积记录"=w355, "error in (no error)"=w359, "要删除的记录"=w348, "数据库引用"=w361) -> ("error out"=w349:errorcluster, "删除量"=w350:dbl, "connection reference out"=w360:T12)  [unwired: 3 in]
        n122 = Merge Errors(w349, w357) -> (w356:errorcluster)
        n123 = case shown="无错误" w349 {
          tunnel: w351 -> [w367 w387]
          tunnel: w348 -> [w362 _]
          tunnel: [w365 w387] -> w347
          tunnel: w350 -> [w364 _]
          frame No Error {
            n124 = Unbundle By Name(w362) -> ("名称"=w368:string)
            n125 = for {
              tunnel: w367 -> [w382] mode=indexing
              tunnel: w368 -> [w385]
              tunnel: [w384] -> w366
              tunnel: [w383] -> w363
              i -> [w384]
              stop <- w383 stop-if-true
              # "找到"
              n126 = Unbundle By Name(w382) -> ("名称"=w386:string)
              n127 = Equal?(x=w386, y=w385) -> (x = y?=w383:bool)
            }
            n128 = case shown="真" w363 {
              tunnel: w367 -> [w369 w373]
              tunnel: w366 -> [_ w372]
              tunnel: [w369 w371] -> w365
              tunnel: w364 -> [_ w370]
              frame False {
                # "没匹配到"
              }
              frame True {
                # "匹配到"
                n129 = in-place {
                  in-place-border: w370 -> [w375]
                  # "替换"
                  n130 = in-place-array #11(w373, w372) -> (w376:T4)
                  n131 = in-place {
                    in-place-border: w375 -> [w381]
                    # "不能减出负数"
                    n132 = in-place-cluster #12(w376) -> ("累积剂量"=w377:dbl)
                    n133 = Subtract(x=w377, y=w381) -> (x-y=w380:dbl)
                    n134 = In Range and Coerce(upper limit=w377, x=w380, lower limit=0.0 ("下限")) -> (coerced(x)=w378:dbl)  [unwired: 1 out]
                    n135 = in-place-cluster #12("累积剂量"=w378) -> (w374:T4)
                  }
                  n136 = in-place-array #11(w374) -> (w371:T4[])  [unwired: 1 out]
                }
              }
            }
          }
          frame Error {
          }
        }
      }
      frame "数据-写改累积记录+改累积剂量" {
        # "即 insert 或 update 累积剂量记录 根据情况判断"
        n137 = Variant To Data(type=T10 {"探头地址与信息"={"网络地址"="", "名称"="", "备注"="", "累积剂量"=0.0, "累积限值"=0.0, "硬件剂量率限值"=enum."一级限值", "剂量率限值1"=0.0, "剂量率限值2"=0.0, "报警方式"=enum."常报警"}, "测量值"={"时间"=timestamp(0 s since 1904-01-01), "数值"=0.0}, "累积记录"={"起始时间"=timestamp(0 s since 1904-01-01), "结束时间"=timestamp(0 s since 1904-01-01), "累积剂量"=0.0}}, Variant=w398) -> (data=w391:T10, error out=w400:errorcluster)  [unwired: 1 in]
        n138 = call "数据表-写入或修改记录.vi"("元素名[]-探测器信息"=w395, "元素名[]-累积记录"=w397, "error in (no error)"=w401, "表名-设备表"=w394, "写改记录数据输入"=w391, "数据库引用"=w403) -> ("error out"=w399:errorcluster, "输出簇"=w389:T10, "累积剂量增量"=w390:dbl, "connection reference out"=w402:T12)  [unwired: 2 in]
        n139 = Merge Errors(w399, w400) -> (w388:errorcluster)
        n140 = case shown="无错误" w388 {
          tunnel: w393 -> [w408 w427]
          tunnel: w391 -> [w410 _]
          tunnel: [w406 w427] -> w392
          tunnel: w390 -> [w405 _]
          frame No Error {
            n141 = Unbundle By Name(w410) -> ("探头地址与信息.网络地址"=w409:string)
            n142 = for {
              tunnel: w408 -> [w422] mode=indexing
              tunnel: w409 -> [w425]
              tunnel: [w424] -> w407
              tunnel: [w423] -> w404
              i -> [w424]
              stop <- w423 stop-if-true
              # "找到"
              n143 = Unbundle By Name(w422) -> ("网络地址"=w426:string)
              n144 = Equal?(x=w426, y=w425) -> (x = y?=w423:bool)
            }
            n145 = case shown="真" w404 {
              tunnel: w408 -> [w411 w415]
              tunnel: w407 -> [_ w414]
              tunnel: [w411 w413] -> w406
              tunnel: w405 -> [_ w412]
              frame False {
                # "没匹配到"
              }
              frame True {
                # "匹配到"
                n146 = in-place {
                  in-place-border: w412 -> [w417]
                  # "替换"
                  n147 = in-place-array #13(w415, w414) -> (w418:T4)
                  n148 = in-place {
                    in-place-border: w417 -> [w421]
                    n149 = in-place-cluster #14(w418) -> ("累积剂量"=w420:dbl)
                    n150 = Add(x=w420, y=w421) -> (x+y=w419:dbl)
                    n151 = in-place-cluster #14("累积剂量"=w419) -> (w416:T4)
                  }
                  n152 = in-place-array #13(w416) -> (w413:T4[])  [unwired: 1 out]
                }
              }
            }
          }
          frame Error {
          }
        }
      }
      frame "读变量-全部设备" {
      }
    }
  }
  "输出数据" <- w3
  "error out" <- w2
